vi "DestroyClone.vi"(8 "error in (no error)":errorcluster, 9 "Exit via Stop Module Req?":bool, 10 "Wait for Module to stop?":bool, 11 "ModuleAdmin":refnum<class "ModuleAdmin.lvclass">) -> (0 "error out":errorcluster, 1 "External Launch":bool, 3 "Mod Admin out":refnum<class "ModuleAdmin.lvclass">)   [LabVIEW 2018, in "ScopePlugins.lvlib"]
uses:
  ScopePlugins.lvlib
  <userlib>/NIST/ModuleAdminLib/ModuleAdmin/ModuleAdmin.lvclass
  C:/Program Files (x86)/National Instruments/LabVIEW 2018/user.lib/NIST/ModuleAdminLib/ModuleAdminBase/ModuleAdminBase.lvclass
  <userlib>/NIST/ModuleAdminLib/ModuleAdmin/ModuleAdmin.lvclass/ModuleAdmin.ctl
  <userlib>/NIST/ModuleAdminLib/ModuleAdmin/Accessors/Read CloneRegRef.vi
  <userlib>/NIST/ModuleAdminLib/CloneRegistration/CloneRegistration.lvclass
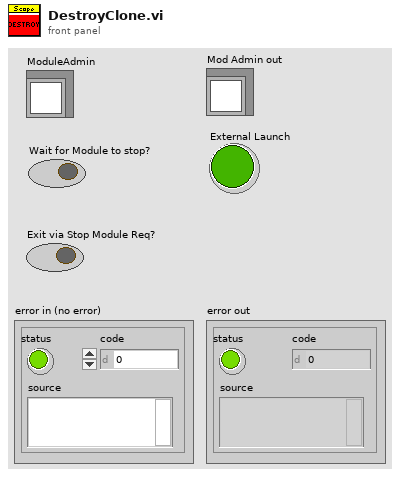
[diagram p1: front panel]
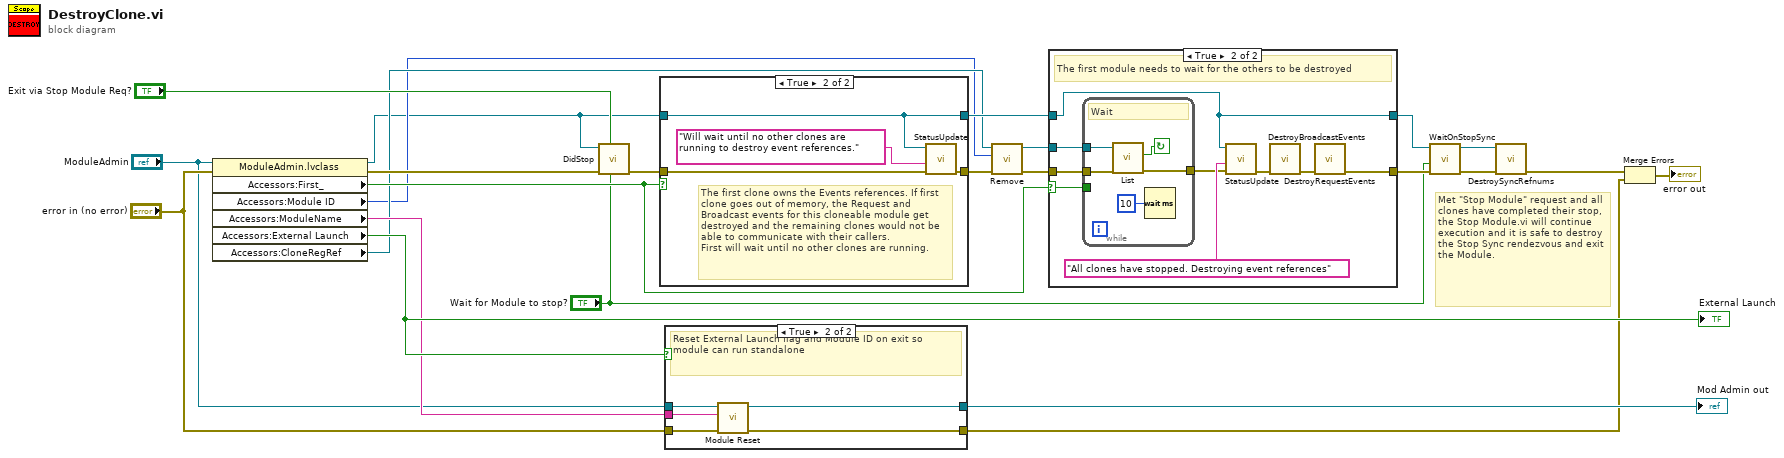
[diagram p0: block diagram]
diagram:
  # "Met \"Stop Module\" request and all clones have completed their stop, the Stop Module.vi will continue execution and it is safe to destroy the Stop Sync rendezvous and exit the Module."
  n1 = property class="ModuleAdmin.lvclass"(reference="ModuleAdmin", error in="error in (no error)") -> (reference out=w3:refnum<class "ModuleAdmin.lvclass">, error out=w24:errorcluster, "Accessors:First_"=w20:bool, "Accessors:Module ID"=w4:i32, "Accessors:ModuleName"=w11:string, "Accessors:External Launch"=w13:bool, "Accessors:CloneRegRef"=w7:refnum<data-value>)
  "External Launch" <- w13
  n2 = call "DidStop.vi"("Wait for Module to stop?"="Wait for Module to stop?", "Exit via Stop Module Req?"="Exit via Stop Module Req?", "error in (no error)"=w24, "ModuleAdmin"=w3) -> ("error out"=w22:errorcluster)  [unwired: 7 in]
  n3 = case shown="True" w20 {
    tunnel: w22 -> [w26 w30]
    tunnel: w3 -> [w25 w27]
    tunnel: [w26 w28] -> w21
    tunnel: [w25 w27] -> w18
    frame False {
    }
    frame True {
      # "The first clone owns the Events references. If first clone goes out of memory, the Request and Broadcast events for this cloneable module get destroyed and the remaining clones would not be able to communicate with their callers.\nFirst will wait until no other clones are running."
      n4 = call "StatusUpdate.vi"("error in (no error)"=w30, "Status"="Will wait until no other clones are running to destroy event references." ("format string"), "ModuleAdmin"=w27) -> ("error out"=w28:errorcluster)  [unwired: 8 in]
    }
  }
  n5 = case shown="True" w13 {
    tunnel: "error in (no error)" -> [w31 w37]
    tunnel: w11 -> [_ w36]
    tunnel: "ModuleAdmin" -> [w32 w35]
    tunnel: [w32 w34] -> w10
    tunnel: [w31 w33] -> w8
    frame False {
    }
    frame True {
      # "Reset External Launch flag and Module ID on exit so module can run standalone"
      n6 = call <userlib>:"Module Reset.vi"("error in (no error)"=w37, "ModuleName"=w36, "Mod Admin in"=w35) -> ("error out"=w33:errorcluster, "Mod Admin out"=w34:refnum<class "ModuleAdmin.lvclass">)  [unwired: 7 in]
    }
  }
  "Mod Admin out" <- w10
  n7 = call <userlib>:"Remove.vi"("error in (no error)"=w21, "Module ID"=w4, "CloneRegRef"=w7) -> ("error out"=w19:errorcluster, "CloneRegRef"=w6:refnum<data-value>)  [unwired: 6 in, 1 out]
  n8 = case shown="True" w20 {
    selector: w20 -> [_ w47]
    tunnel: w19 -> [w38 w48]
    tunnel: w18 -> [w39 w40]
    tunnel: [w38 w42] -> w17
    tunnel: [w39 w40] -> w2
    tunnel: w6 -> [_ w41]
    frame False {
    }
    frame True {
      # "The first module needs to wait for the others to be destroyed"
      n9 = while {
        tunnel: w48 -> [w53]
        tunnel: w47 -> [_]
        tunnel: [w52] -> w45
        tunnel: w41 -> [w49]
        stop <- w51 continue-if-true
        # "Wait"
        n10 = call <userlib>:"List.vi"("error in (no error)"=w53, "CloneRegRef"=w49) -> ("error out"=w52:errorcluster, "Found?"=w51:bool)  [unwired: 4 in, 4 out]
        n11 = Wait (ms)(milliseconds to wait=u32 10) -> ()  [unwired: 1 out]
      }
      n12 = call "StatusUpdate.vi"("error in (no error)"=w45, "Status"="All clones have stopped. Destroying event references", "ModuleAdmin"=w40) -> ("error out"=w44:errorcluster)  [unwired: 8 in]
      n13 = call "DestroyBroadcastEvents.vi"("error in (no error)"=w44) -> ("error out"=w43:errorcluster)  [unwired: 10 in]
      n14 = call "DestroyRequestEvents.vi"("error in (no error)"=w43) -> ("error out"=w42:errorcluster)  [unwired: 10 in]
    }
  }
  n15 = call <userlib>:"WaitOnStopSync.vi"("error in (no error)"=w17, "WaitForModuleToStop?"="Wait for Module to stop?", "ModuleAdmin"=w2) -> ("error out"=w15:errorcluster, "ModuleAdmin"=w1:refnum<class "ModuleAdmin.lvclass">)  [unwired: 7 in]
  n16 = call <userlib>:"DestroySyncRefnums.vi"("error in (no error)"=w15, "ModuleAdmin"=w1) -> ("error out"=w14:errorcluster)  [unwired: 9 in]
  n17 = Merge Errors(w14, w8) -> (→"error out":errorcluster)
